vi "RegisterUserEvent.vi"(8 "error in":errorcluster, 11 "message ref in":refnum<class "CLM_LocalMessage_UserEvent.lvclass">) -> (0 "error out":errorcluster, 3 "message ref out":refnum<class "CLM_LocalMessage_UserEvent.lvclass">)   [LabVIEW 2013, in "CLM_LocalMessage_UserEvent.lvclass"]
uses:
  CLM_LocalMessage_UserEvent.lvclass
  CLM_LocalMessage_UserEvent.lvclass/CLM_LocalMessage_UserEvent.ctl
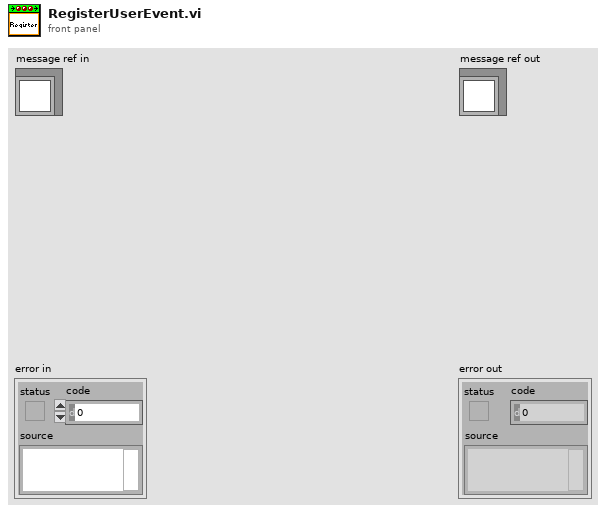
[diagram p1: front panel]
types:
  T1 = typedef "CLM_LocalMessage_UserEvent.lvclass/MessageUserEvent.ctl" = refnum<user-event>
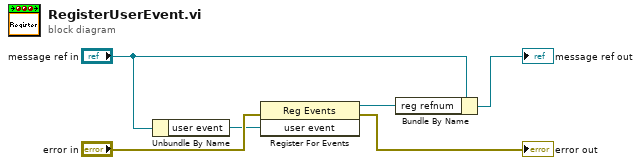
[diagram p0: block diagram]
diagram:
  n1 = Unbundle By Name("message ref in") -> ("user event"=w1:T1)
  n2 = register-events(error in="error in", w1) -> (reference out=w2:refnum<event-registration>, error out=→"error out":errorcluster)  [unwired: 1 in]
  n3 = Bundle By Name(cluster="message ref in", "reg refnum"=w2) -> (→"message ref out":refnum<class "CLM_LocalMessage_UserEvent.lvclass">)
